vi "TESTER (point clicked on graph).vi"() -> ()   [LabVIEW 2009]
uses:
  <vilib>/Utility/miscctls.llb/LVPoint32TypeDef.ctl
panel:
  in  "stop":bool
  out "mouse coords":T1
  out "Point clicked":cluster{"x":dbl, "y":dbl}
  out "Valid mouse position":bool
  out "XY Graph":cluster{dbl[], "Best Cubic Spline Fit":dbl[]}(graph)
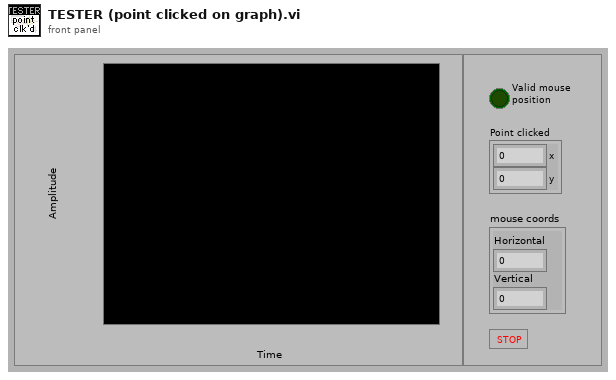
[diagram p1: front panel]
types:
  T1 = typedef "LVPoint32TypeDef.ctl" = cluster{"Horizontal":i32, "Vertical":i32}
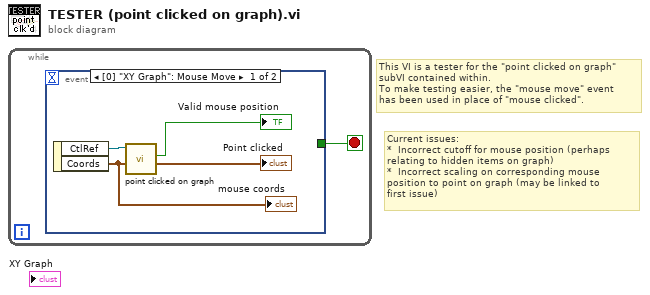
[diagram p0: block diagram]
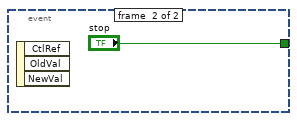
[diagram p2: hidden frame]
diagram:
  # "Current issues:\n*  Incorrect cutoff for mouse position (perhaps\nrelating to hidden items on graph)\n*  Incorrect scaling on corresponding mouse\nposition to point on graph (may be linked to \nfirst issue)"
  # "This VI is a tester for the \"point clicked on graph\"\nsubVI contained within.\nTo make testing easier, the \"mouse move\" event\nhas been used in place of \"mouse clicked\"."
  n1 = while {
    stop <- w1 stop-if-true
    n2 = event shown="[0] \"XY Graph\": Mouse Move" {
      selector: _ -> [_ _]
      dyn-events: _ -> [_ _]
      timeout: _ -> [_ _]
      tunnel: [_ "stop"] -> w1
      event #0 {
        n3 = event-data() -> ("CtlRef"=w3:refnum<vi>, "Coords"=w2:T1)  [unwired: 1 in]
        "mouse coords" <- w2
        n4 = call "point clicked on graph.vi"("Mouse Position"=w2, "Graphchart reference"=w3) -> ("Point clicked"=→"Point clicked":cluster{"x":dbl, "y":dbl}, "Valid mouse position"=→"Valid mouse position":bool)  [unwired: 8 in]
      }
      event #1 {
        n5 = event-data() -> ()  [unwired: 1 in, 3 out]
      }
    }
  }
